vi "Set Enable Debugging.vi"(8 "error in (no error)":errorcluster, 9 "Wait for debugger on launch (false)":bool, 10 "Enable debugging (false)":bool, 11 "NI_AB_API_Application in":refnum<class "NI_AB_API_Application.lvclass">) -> (0 "error out":errorcluster, 3 "NI_AB_API_Application out":refnum<class "NI_AB_API_Application.lvclass">)   [LabVIEW 2020, in "NI_AB_API_Application.lvclass"]
uses:
  <vilib>/AppBuilder/AB_API/Application/NI_AB_API_Application.lvclass
  <vilib>/AppBuilder/AB_API/Application/NI_AB_API_Application.lvclass/NI_AB_API_Application.ctl
  <vilib>/AppBuilder/AB_Classes/Application/AB_Application.lvclass
  <vilib>/AppBuilder/AB_API/Build/NI_AB_API_Build.lvclass
  <vilib>/AppBuilder/AB_API/Targetfile/NI_AB_API_Targetfile.lvclass
  e:/builds/penguin/labview/branches/2020/dev/dist/vi.lib/AppBuilder/AB_API/Targetfile/NI_AB_API_Targetfile.lvclass
  e:/builds/penguin/labview/branches/2020/dev/dist/vi.lib/AppBuilder/AB_API/Build/NI_AB_API_Build.lvclass
  e:/builds/penguin/labview/branches/2020/dev/dist/vi.lib/AppBuilder/AB_API/Application/NI_AB_API_Application.lvclass
  e:/builds/penguin/labview/branches/2020/dev/dist/vi.lib/AppBuilder/AB_Classes/TargetFile/AB_Targetfile.lvclass
  e:/builds/penguin/labview/branches/2020/dev/dist/vi.lib/AppBuilder/AB_Classes/Build/AB_Build.lvclass
  e:/builds/penguin/labview/branches/2020/dev/dist/vi.lib/AppBuilder/AB_Classes/Application/AB_Application.lvclass
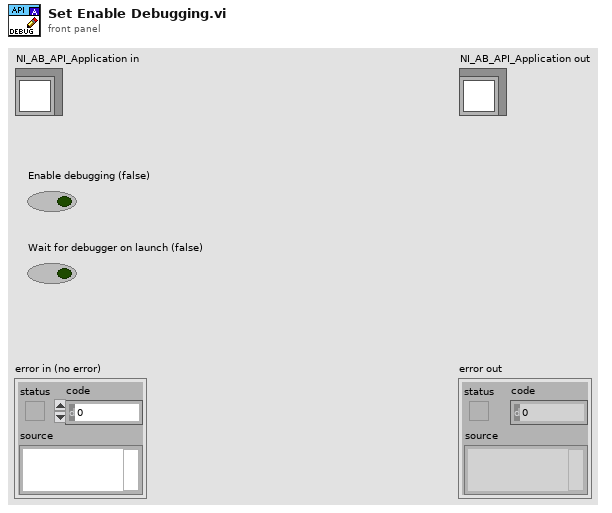
[diagram p1: front panel]
types:
  T1 = typedef "AB_Application.ctl" = cluster{"INI_path":path, "INI_itemID":string, "INI_GUID":string, "aliasPath":path, "aliasItemID":string, "aliasGUID":string, "waitDebugging":bool, "copyErrors":bool, "useFFRTE":bool, "includeHWConfig":bool, "showHWConfig":bool, "winsec.certificate":string, "winsec.timestamp":string, "winsec.description":string, "winsec.manifestItemID":string, "winsec.manifestPath":path, "web service itemIDs":string[], "Embedded Server Configuration":T2, "Server Type":enum32{"NI Web Server", "Application Web Server"}}
  T2 = typedef "AB_Embedded_Server_Configuration.ctl" = cluster{"HTTP enabled?":bool, "HTTP port":i32, "HTTPS enabled?":bool, "HTTPS port":i32, "SSL certificate file":path}
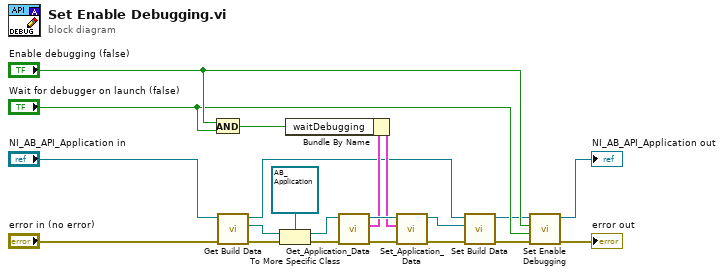
[diagram p0: block diagram]
diagram:
  n1 = And(x="Enable debugging (false)", y="Wait for debugger on launch (false)") -> (x .and. y?=w12:bool)
  n2 = call <vilib>:"Get Build Data.vi"("error in (no error)"="error in (no error)", "NI_AB_API_Build in"="NI_AB_API_Application in") -> ("error out"=w4:errorcluster, "AB_Build.lvclass"=w7:refnum<class "AB_Build.lvclass">, "NI_AB_API_Build out"=w11:refnum<class "NI_AB_API_Application.lvclass">)  [unwired: 7 in]
  n3 = To More Specific Class(target class=refnum<class "AB_Application.lvclass"> refnum ("AB_Application in"), reference=w7, error in=w4) -> (specific class reference=w6:refnum<class "AB_Application.lvclass">, error out=w3:errorcluster)
  n4 = call <vilib>:"Get_Application_Data.vi"("error in (no error)"=w3, "AB_Application in"=w6) -> ("error out"=w2:errorcluster, "data"=w14:T1, "AB_Application out"=w15:refnum<class "AB_Application.lvclass">)  [unwired: 7 out]
  n5 = Bundle By Name(cluster=w14, "waitDebugging"=w12) -> (w13:T1)
  n6 = call <vilib>:"Set_Application_Data.vi"("error in (no error)"=w2, "data"=w13, "Class in"=w15) -> ("error out"=w1:errorcluster, "Class out"=w9:refnum<class "AB_Application.lvclass">)  [unwired: 7 out]
  n7 = call <vilib>:"Set Build Data.vi"("error in (no error)"=w1, "AB_Build.lvclass"=w9, "NI_AB_API_Build in"=w11) -> ("error out"=w8:errorcluster, "NI_AB_API_Build out"=w10:refnum<class "NI_AB_API_Application.lvclass">)  [unwired: 7 in]
  n8 = call-parent "Set Enable Debugging.vi"("error in (no error)"=w8, "Wait for debugger on launch (false)"="Wait for debugger on launch (false)", "Enable debugging (false)"="Enable debugging (false)", "NI_AB_API_Targetfile in"=w10) -> ("error out"=→"error out":errorcluster, "NI_AB_API_Targetfile out"=→"NI_AB_API_Application out":refnum<class "NI_AB_API_Application.lvclass">)  [unwired: 6 in]
